vi "Initialize-parser.vi"(8 "error in (no error)":errorcluster, 10 "Main VI ref":refnum<vi>, 11 "Data ref. in":T1) -> (0 "error out":errorcluster, 3 "Data ref.":T1)   [LabVIEW 2013, in "HardwareCharacterization.lvlib" / "HC-Main.lvclass"]
uses:
  HC-Main.lvclass
  Object-reference.ctl
  HC-Main.lvclass/HC-Main.ctl
  ScanParser/HC-ScanParser.lvclass
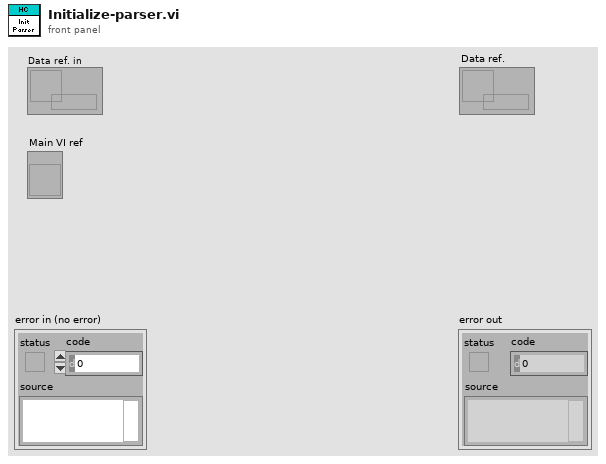
[diagram p1: front panel]
types:
  T1 = typedef "HardwareCharacterization.lvlib/HC-Main.lvclass/Object-reference.ctl" = refnum<data-value>
  T2 = typedef "HardwareCharacterization.lvlib/HC-ScanParser.lvclass/Object-reference.ctl" = refnum<data-value>
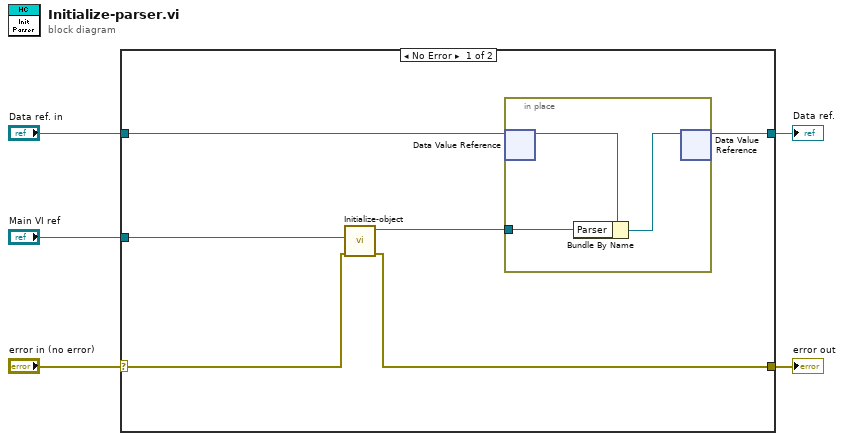
[diagram p0: block diagram]
diagram:
  n1 = case shown="No Error" "error in (no error)" {
    selector: "error in (no error)" -> [w7 w16]
    tunnel: [w6 w16] -> w4
    tunnel: "Data ref. in" -> [w10 w15]
    tunnel: [w11 w15] -> w2
    tunnel: "Main VI ref" -> [w8 _]
    frame No Error {
      n2 = call "Initialize-object.vi"("error in (no error)"=w7, "VI Reference"=w8) -> ("error out"=w6:errorcluster, "Reference out"=w9:T2)  [unwired: 8 in]
      n3 = in-place {
        in-place-border: w9 -> [w14]
        n4 = in-place-dvr #1(w10) -> (w12:refnum<class "HC-Main.lvclass">)  [unwired: 1 out]
        n5 = Bundle By Name(cluster=w12, "Parser"=w14) -> (w13:refnum<class "HC-Main.lvclass">)
        n6 = in-place-dvr #1(w13) -> (w11:T1)  [unwired: 1 out]
      }
    }
    frame Error {
    }
  }
  "error out" <- w4
  "Data ref." <- w2
